vi "Read Initial Air Mass.vi"(8 "error in (no error)":errorcluster, 11 "TCS in":refnum<class "TCS.lvclass">) -> (0 "error out":errorcluster, 2 "Initial Air Mass":string, 3 "TCS out":refnum<class "TCS.lvclass">)   [LabVIEW 2018, in "TCS.lvclass"]
uses:
  TCS.lvclass
  TCS.lvclass/TCS.ctl
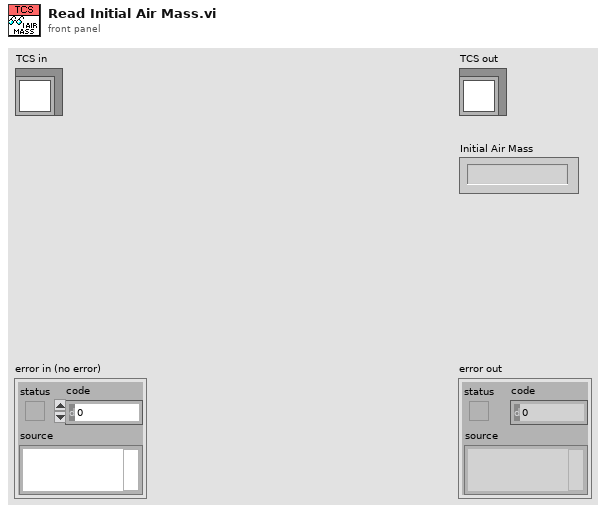
[diagram p1: front panel]
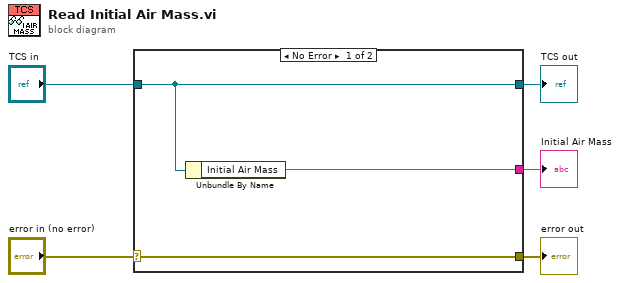
[diagram p0: block diagram]
diagram:
  n1 = case shown="No Error" "error in (no error)" {
    selector: "error in (no error)" -> [w8 w9]
    tunnel: [w8 w9] -> w4
    tunnel: [w7 w10] -> w2
    tunnel: "TCS in" -> [w7 w10]
    tunnel: [w6 _] -> w1
    frame No Error {
      n2 = Unbundle By Name(w7) -> ("Initial Air Mass"=w6:string)
    }
    frame Error {
    }
  }
  "error out" <- w4
  "TCS out" <- w2
  "Initial Air Mass" <- w1
